vi "Identify.vi"(8 "error in (no error)":errorcluster, 11 "Skyworks - 2G PVT in":refnum<class "Skyworks - 2G PVT.lvclass">) -> (0 "error out":errorcluster, 2 "Plugin is Valid":bool, 3 "Skyworks - 2G PVT out":refnum<class "Skyworks - 2G PVT.lvclass">)   [LabVIEW 2016, in "Skyworks - 2G PVT.lvlib" / "Skyworks - 2G PVT.lvclass"]
uses:
  Skyworks - 2G PVT.lvclass
  C:/Sequence Automation/Plugins/Measurement Interface.lvlibp/Measurement Interface.lvclass
  C:/Sequence Automation/Plugins/Measurements/Skyworks - PVT.lvlibp/Skyworks - PVT.lvclass
  Plugins/Measurement Interface.lvlibp/Private Methods/Measurement Definition Entry/Read Measurement Definition Entry.vi
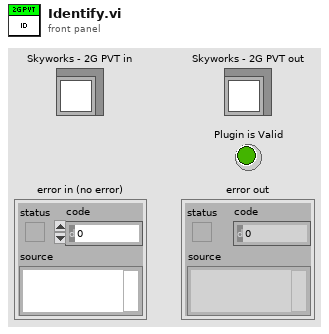
[diagram p1: front panel]
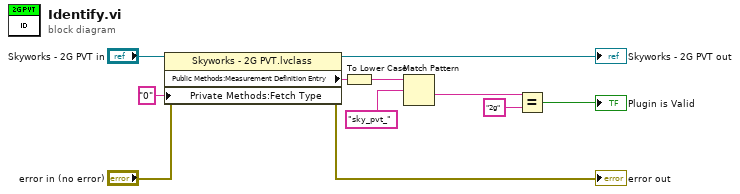
[diagram p0: block diagram]
diagram:
  n1 = property class="Skyworks - 2G PVT.lvclass"(reference="Skyworks - 2G PVT in", error in="error in (no error)", "Private Methods:Fetch Type"="0" ("Fetch Type")) -> (reference out=→"Skyworks - 2G PVT out":refnum<class "Skyworks - 2G PVT.lvclass">, error out=→"error out":errorcluster, "Public Methods:Measurement Definition Entry"=w10:string)
  n2 = To Lower Case(string=w10) -> (all lower case string=w8:string)
  n3 = Match Pattern(string=w8, regular expression="sky_pvt_") -> (after substring=w7:string)  [unwired: 1 in, 3 out]
  n4 = Equal?(x=w7, y="2g") -> (x = y?=→"Plugin is Valid":bool)
